vi "Get Assets.vi"(8 "Error In":errorcluster, 10 "Asset ID":string, 11 "Session In":refnum<class "NI Skyline Configuration HTTP.lvclass">) -> (0 "Error Out":errorcluster, 2 "Asset":T1, 3 "Session Out":refnum<class "NI Skyline Configuration HTTP.lvclass">)   [LabVIEW 2020]
uses:
  <vilib>/Skyline/Configuration/Configuration HTTP_class/NI Skyline Configuration HTTP.lvclass
  <vilib>/Skyline/Configuration/Configuration HTTP_class/NI Skyline Configuration HTTP.lvclass/NI Skyline Configuration HTTP.ctl
  <vilib>/Skyline/Configuration/Configuration HTTP_class/Read Server URL.vi
  <vilib>/httpClient/LabVIEWHTTPClient.lvlib
  <vilib>/addons/_JKI.lib/Serialization/JSON/JKI JSON Serialization.lvlib
panel:
  out "Server URL":string
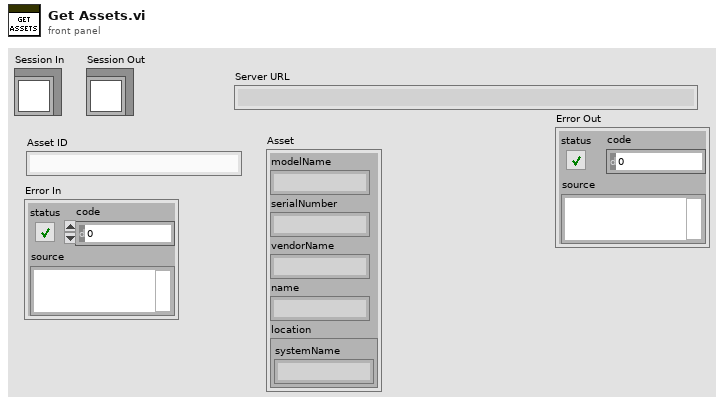
[diagram p1: front panel]
types:
  T1 = cluster{"modelName":string, "serialNumber":string, "vendorName":string, "name":string, "location":cluster{"systemName":string}}
  T2 = typedef "LabVIEWHTTPClient.lvlib/ClientHandle.ctl" = refnum<k1>
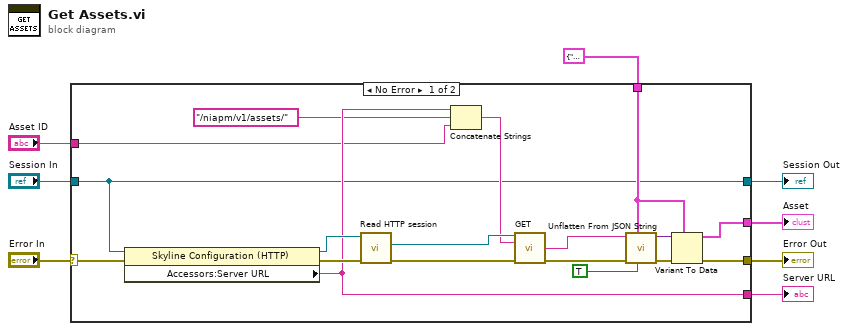
[diagram p0: block diagram]
diagram:
  n1 = case shown="No Error" "Error In" {
    selector: "Error In" -> [w10 w27]
    tunnel: [w22 _] -> w8
    tunnel: "Session In" -> [w9 w28]
    tunnel: "Asset ID" -> [w16 _]
    tunnel: [w14 w27] -> w5
    tunnel: T1 {"modelName"="", "serialNumber"="", "vendorName"="", "name"="", "location"={"systemName"=""}} ("asset") -> [w12 _]
    tunnel: [w11 _] -> w3
    tunnel: [w9 w28] -> w1
    frame No Error {
      n2 = property class="Skyline Configuration (HTTP)"(reference=w9, error in=w10) -> (reference out=w25:refnum<class "NI Skyline Configuration HTTP.lvclass">, error out=w24:errorcluster, "Accessors:Server URL"=w22:string)
      n3 = call <vilib>:"Read HTTP session.vi"("error in (no error)"=w24, "HTTP configuration in"=w25) -> ("error out"=w23:errorcluster, "http session"=w26:T2)  [unwired: 7 in, 1 out]
      n4 = Concatenate Strings(w22, "/niapm/v1/assets/" ("string"), w16) -> (w21:string)
      n5 = call <vilib>:"GET.vi"("client handle"=w26, "url"=w21, "error in (no error)"=w23) -> ("body"=w19:string, "error out"=w17:errorcluster)  [unwired: 9 in, 2 out]
      n6 = call <vilib>:"Unflatten From JSON String.vi"("Nulls as Defaults (F)"=TRUE ("default null elements? (F)"), "Type and Defaults"=w12, "error in (no error)"=w17, "JSON String"=w19) -> ("error out"=w15:errorcluster, "Variant"=w13:variant)  [unwired: 6 in]
      n7 = Variant To Data(error in=w15, type=w12, Variant=w13) -> (data=w11:T1, error out=w14:errorcluster)
    }
    frame Error {
    }
  }
  "Server URL" <- w8
  "Error Out" <- w5
  "Session Out" <- w1
  "Asset" <- w3
